vi "Drive Controller.vi"(8 "error in":errorcluster) -> ()   [LabVIEW 2018]
doc: "This VI executes continuously carrying out the current operation and responding to updates or new operation requests. It will often contain the timing or control code that is difficult to place directly in TeleOp. This VI generally opens all sensors and motors and isolates the rest of the robot code from knowing implementation details of how the operations are carried out."
uses:
  <vilib>/Rock Robotics/WPI/Framework/Completion Status.ctl
  Drive Setpoints.ctl
  Drive Operations.ctl
  <vilib>/Rock Robotics/WPI/ThirdParty/REV Robotics/SPARK MAX/Typedef/Spark MAX Control Type.ctl
  <vilib>/Rock Robotics/WPI/Gyro/WPI_GyroDevRef.ctl
  <vilib>/Rock Robotics/SystemInterfaces/AI/FPGA_AIChannel.ctl
  <vilib>/Rock Robotics/SystemInterfaces/spilib/spi_bus.ctl
  CAN Functions/SPARKMAX6Motor.ctl
  <vilib>/Rock Robotics/WPI/MotorControl/WPI_MotorControlDeviceRef.ctl
  <vilib>/Rock Robotics/WPI/MotorControl/WPI_MotorControlType.ctl
  <vilib>/Rock Robotics/SystemInterfaces/DIO/FPGA_DIOPWMChannel.ctl
  <vilib>/Rock Robotics/WPI/PWM/WPI_PWMDeadband.ctl
  <vilib>/Rock Robotics/SystemInterfaces/DIO/FPGA_DIOChannel.ctl
  <vilib>/Platform/TimedLoop/XDataNode/timing_clust.ctl
  <vilib>/Platform/TimedLoop/XDataNode/nitl_modes.ctl
  <vilib>/Platform/TimedLoop/XDataNode/wakeup.ctl
  Odometry/Typedef/Odometry.ctl
  Odometry/Typedef/Velocity Data.ctl
  <vilib>/Rock Robotics/WPI/ThirdParty/Phoenix-LabVIEW/Motor Controller/Controls/CTRE_Phoenix_MotorControl_ControlMode.ctl
  Pure Pursuit/Typedef/Pure Pursuit Telemetry.ctl
  Pure Pursuit/Typedef/Path Point.ctl
  Is High Gear.vi
  <vilib>/platform/TimedLoop/XDataNode/XDataNode.xnode
  <vilib>/Platform/TimedLoop/XDataNode/XDNodeRunTimeDep.lvlib
  <vilib>/ptbypt/NI_PtbyPt.lvlib
  Pure Pursuit/Pure Pursuit.lvlib
  <vilib>/Analysis/NI_AALPro.lvlib
panel:
  in  "Control Mode":T1
  in  "Tab Control":T2(tab)=enum."Settings"
  in  "Interactive Values":T3
  out "Setpoints":T5(graph)={"Don't move motors while reserved"=0.0, "Don't move motors while reserved"=0.0, "Left Velocity Raw"=0.0, "Right Velocity Raw"=-0.0, 0.0}
  in  "Buttons":cluster{"Execute Cmd":bool, "Abort Cmd":bool}
  out "Command Timing":cluster{"Start Time (ms)":u32, "Iterations":i32}={"Start Time (ms)"=2524017, "Iterations"=0}
  out "Status":T6
  in  "PID Constants Drivetrain":T7={"P Gain"=0.00656, "I Gain"=0.0, "D Gain"=0.01313, "F Gain"=0.005515, "I Zone"=0.0, "Min Output"=-1.0, "Max Output"=1.0} {"Max Output" min=-1.0 max=1.0 step=0.01; "Min Output" min=-1.0 max=1.0 step=0.01; "I Zone" step=0.01; "F Gain" step=0.01; "D Gain" step=0.01; "I Gain" step=0.01; "P Gain" min=0.0 step=0.01}
  in  "PIDF gains":cluster{"Kp":dbl, "Ki":dbl, "Kd":dbl, "Kf":dbl}={"Kp"=7.5, "Ki"=0.05, "Kd"=2.5, "Kf"=0.0} caption="PIDF gains (turn to angle only)" {"Kf" format="%.3f"; "Kd" format="%.5f"; "Ki" format="%.5f"; "Kp" format="%.5f"}
  in  "i Zone":dbl=8.0 format="%.2f"
  in  "Trackwidth":dbl=25.0 format="%#_13g"
  in  "Max Velocity":dbl=110.0
  in  "Max Accel":dbl=210.0
  in  "Lookahead":dbl=19.0
  in  "kffv":dbl
  in  "kffa":dbl=0.05
  in  "Velocity Offset High Gear":dbl
  in  "Velocity Offset Low Gear":dbl=0.08
  in  "Value":dbl
  in  "Run":bool
  out "Waveform Chart":dbl(graph)
  out "XY Graph":cluster{"X":dbl, "Y":dbl}[](graph)
  in  "Test":string(combo)="quasi-static ramp"
  out "Path":cluster{dbl[], dbl[]}[](graph)
  in  "Points to Follow":cluster{dbl[], dbl[]}={[0.0, 40.0, 60.0, 100.0], [0.0, 20.0, 80.0, 40.0]}
  in  "Type of Interpolation":T8(ring)=enum."Spline"
  in  "Interpolation factor (n)":i32(slide)=100 scale=0.0..20.0
  in  "Build and set Path":bool
  out "Left and Right Motor Values":T9(graph)
  out "Process Variable Vs. Setpoint":cluster{dbl, "setpoint":dbl}(graph)
  in  "PIDF gains":cluster{"Kp":dbl, "Ki":dbl, "Kd":dbl, "Kf":dbl}={"Kp"=0.06, "Ki"=0.0, "Kd"=0.0, "Kf"=0.0} {"Kf" format="%.3f"; "Kd" format="%.3f"; "Ki" format="%.3f"; "Kp" format="%.3f"}
  in  "output range 2":cluster{"output high":dbl, "output low":dbl}={"output high"=0.6, "output low"=-0.6} {"output low" format="%.2f"; "output high" format="%.2f"}
  in  "i Zone":dbl format="%.2f"
  in  "Allowed Error":dbl
  out "Current\nCmd":string="Started at  20:49:40.426\nDefault: Reserve,  L 0.0, R 0.0, D 0.000000"
  # "Click here to set min"
  # "Interactive Command: You may fill in the settings for a command\nand schedule it with the Execute button. You can observe and abort\nany command while fine tuning the code for the controller."
  # "Pure Pursuit"
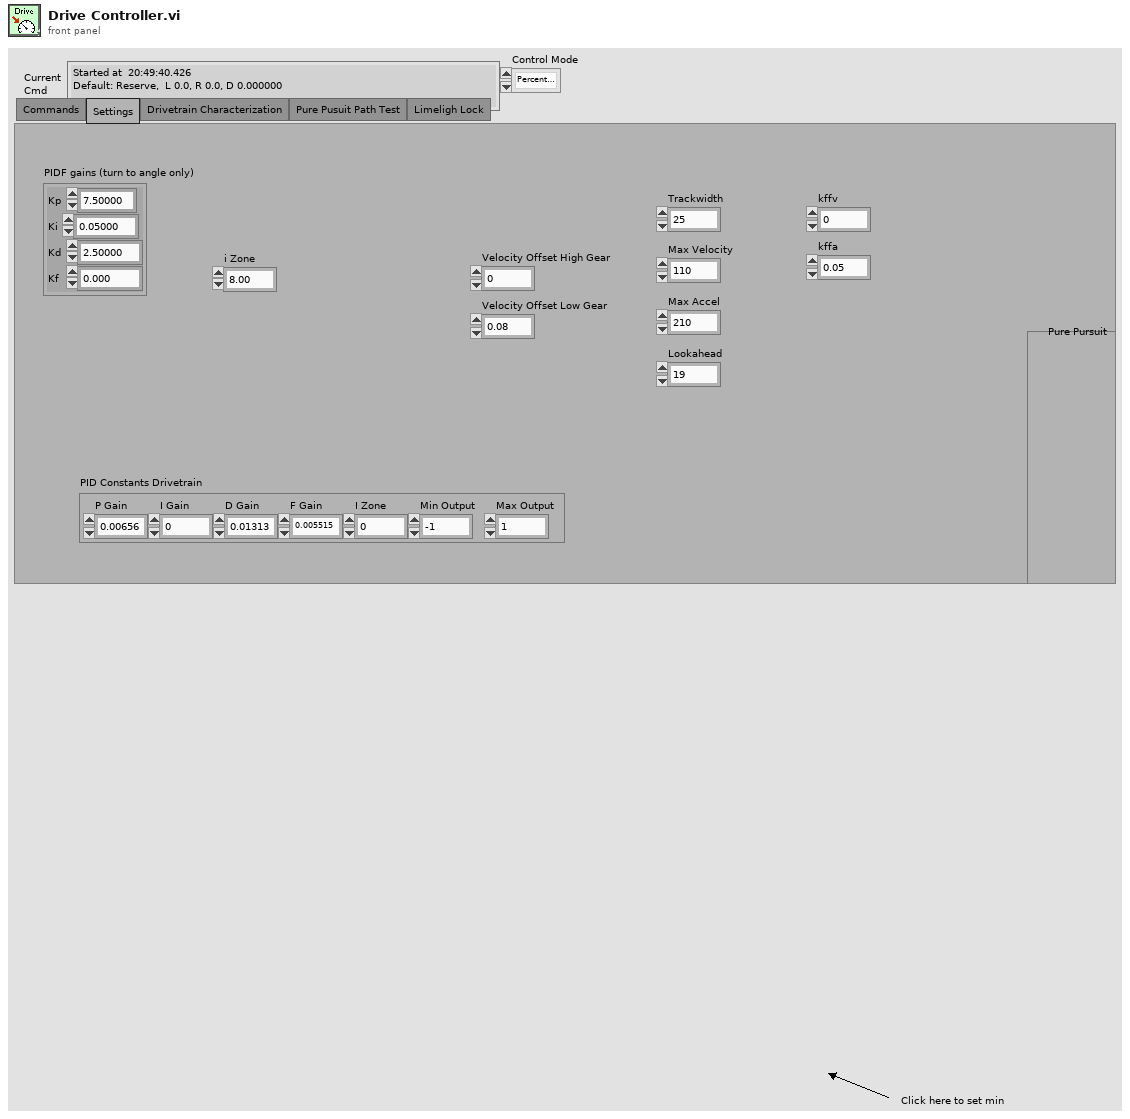
[diagram p1: front panel]
types:
  T1 = typedef "Spark MAX Control Type.ctl" = enum16{"Percent VBus", "Voltage", "Velocity", "Position", "Smart Motion", "Current", "Smart Velocity"}
  T2 = enum32{"Commands", "Settings", "Drivetrain Characterization", "Pure Pusuit Path Test", "Limeligh Lock"}
  T3 = typedef "Drive Setpoints.ctl" = cluster{"Operation":T4, "Left Setpoint":dbl, "Right Setpoint":dbl, "Duration":dbl, "Data":variant}
  T4 = typedef "Drive Operations.ctl" = enum16{"Reserve", "Read Current", "Immediate", "Drive for Time", "Drive for Distance", "Turn to Angle", "Drivetrain Char", "Pure Pursuit", "Limelight Lock"}
  T5 = cluster{"Don't move motors while reserved":dbl, "Don't move motors while reserved":dbl, "Left Velocity Raw":sgl, "Right Velocity Raw":sgl, sgl}
  T6 = typedef "Completion Status.ctl" = enum16{"Successful", "Aborted", "Incomplete"}
  T7 = cluster{"P Gain":dbl, "I Gain":dbl, "D Gain":dbl, "F Gain":dbl, "I Zone":dbl, "Min Output":dbl, "Max Output":dbl}
  T8 = enum16{"Linear", "Polynomial", "Spline", "Rational"}
  T9 = cluster{"Left Motor Value":dbl, "Right Motor Value":dbl}
  T10 = typedef "WPI_GyroDevRef.ctl" = cluster{"DevStatus":errorcluster, "Analog Channel":T11, "Gain (VoltsPerDegree/Second)":dbl, "Gyro Type":enum16{"Analog", "XRS450"}, "Handle":i32, "SPI Bus":T12, "Device Found":bool, "Sample Rate":dbl, "Calibrate On Open":bool, "Offset":dbl}
  T11 = typedef "FPGA_AIChannel.ctl" = enum8{"AI 0", "AI 1", "AI 2", "AI 3", "AI MXP 0", "AI MXP 1", "AI MXP 2", "AI MXP 3", "Invalid"}
  T12 = typedef "spi_bus.ctl" = enum16{"SPI On-Board, CS0", "SPI On-Board, CS1", "SPI On-Board, CS2", "SPI On-Board, CS3", "SPI MXP", "Invalid"}
  T13 = typedef "SPARKMAX6Motor.ctl" = cluster{"FrontLeftMaster":T14, "FrontLeftSlave1":T14, "FrontLeftSlave2":T14, "FrontRightMaster":T14, "FrontRightSlave1":T14, "FrontRightSlave2":T14}
  T14 = typedef "WPI_MotorControlDeviceRef.ctl" = cluster{"DeviceStatus":errorcluster, "Type":T15, "PWM":cluster{"PWM Channel":T16, "DeadBand":T17}, "CAN":cluster{"Device Number":u8, "SetOutput VI Ref":variant, "GetOutput VI Ref":variant, "Enable VI Ref":variant, "Disable VI Ref":variant, "Data":variant}, "Invert":bool, "DIO PWM":cluster{"PWM \"Enable\" Channel":T16, "DIOChannel":T18, "PWM Rate":dbl}}
  T15 = typedef "WPI_MotorControlType.ctl" = enum16{"PWM", "CAN", "DIO PWM"}
  T16 = typedef "FPGA_DIOPWMChannel.ctl" = enum8{"PWM 0", "PWM 1", "PWM 2", "PWM 3", "PWM 4", "PWM 5", "PWM 6", "PWM 7", "PWM 8", "PWM 9", "PWM MXP 0", "PWM MXP 1", "PWM MXP 2", "PWM MXP 3", "PWM MXP 4", "PWM MXP 5", "PWM MXP 6", "PWM MXP 7", "PWM MXP 8", "PWM MXP 9", "Invalid"}
  T17 = typedef "WPI_PWMDeadband.ctl" = cluster{"Name":string, "maxPositivePwm":i32, "minPositivePwm":i32, "centerPwm":i32, "maxNegativePwm":i32, "minNegativePwm":i32, "angularRange":u16}
  T18 = typedef "FPGA_DIOChannel.ctl" = enum8{"DIO 0", "DIO 1", "DIO 2", "DIO 3", "DIO 4", "DIO 5", "DIO 6", "DIO 7", "DIO 8", "DIO 9", "DIO MXP 0", "DIO MXP 1", "DIO MXP 2", "DIO MXP 3", "DIO MXP 4", "DIO MXP 5", "DIO MXP 6", "DIO MXP 7", "DIO MXP 8", "DIO MXP 9", "DIO MXP 10", "DIO MXP 11", "DIO MXP 12", "DIO MXP 13", "DIO MXP 14", "DIO MXP 15", "SPI Port CS1", "SPI Port CS2", "SPI Port CS3", "SPI Port MISO", "SPI Port MOSI", "Invalid"}
  T19 = typedef "XDNodeRunTimeDep.lvlib/timing_clust.ctl" = cluster{"Expected End [f-1]":u64, "Actual End [f-1]":u64, "Finished Late? [f-1]":bool, "Expected End [i-1]":u64, "Actual End [i-1]":u64, "Finished Late? [i-1]":bool, "Expected Start [i]":u64, "Actual Start [i]":u64, "Expected Start [f]":u64, "Actual Start [f]":u64, "Source Name":string, "Structure Name":string, "Period":i64, "Deadline":i64, "Offset":i64, "Start":i64, "Priority":i32, "Timeout":i32, "Mode":T20, "Wakeup Reason":T21, "Error":errorcluster, "Source Type":string, "Secondary Source Type":string, "Global End Time":u64, "Global Start Time":u64, "Frame Duration":u64, "Iteration Duration":u64, "Assigned CPU":i32, "I/O Scan Engine Mode":u32}
  T20 = typedef "XDNodeRunTimeDep.lvlib/nitl_modes.ctl" = enum32{"No Change", "Process missed periods, maintain original phase", "Discard missed periods, maintain original phase", "Process missed periods, ignore original phase", "Discard missed periods, ignore original phase"}
  T21 = typedef "XDNodeRunTimeDep.lvlib/wakeup.ctl" = enum32{"Normal", "Aborted", "Asynchronous wakeup", "Timing source error", "Timed loop error", "Timeout"}
  T22 = typedef "Command Status Info.ctl" = cluster{"Name":string, "Status":T6, "notifier out":T23}
  T23 = typedef "Completion Notifier.ctl" = refnum<notifier>
  T24 = cluster{"SubSystem Data":T3, cluster{"Start Time (ms)":u32, "Iterations":i32}, cluster{"Command Info":T22, "Description":string, "Default Command":T3, "queue out":refnum<queue>, "Subsystem Name":string}}
  T25 = typedef "Pure Pursuit.lvlib/Pure Pursuit Telemetry.ctl" = cluster{"Target Point":T26, "Close Point":T26, "Curvature":dbl, "index out":i32}
  T26 = typedef "Pure Pursuit.lvlib/Path Point.ctl" = cluster{"x":dbl, "y":dbl, "heading":dbl, "curvature":dbl, "total distance":dbl, "velocity expected":dbl}
  T27 = typedef "Odometry.ctl" = cluster{"x":dbl, "y":dbl, "theta":dbl, "Left Encoder":dbl, "Right Encoder":dbl, "Late Iterations":i16}
  T28 = typedef "CTRE_Phoenix_MotorControl_ControlMode.ctl" = u16
  T29 = typedef "Velocity Data.ctl" = cluster{"Right Velocity Raw":sgl, "Left Velocity Raw":sgl}
  T30 = cluster{"SubSystem Data":T3, cluster{"Start Time (ms)":u32, "Iterations":i32}, "Default Command Arguments":cluster{"Command Info":T22, "Description":string, "Default Command":T3, "queue out":refnum<queue>, "Subsystem Name":string}}
  T31 = cluster{"P Gain":bool, "I Gain":bool, "D Gain":bool, "F Gain":bool, "I Zone":bool, "Min Output":bool, "Max Output":bool}
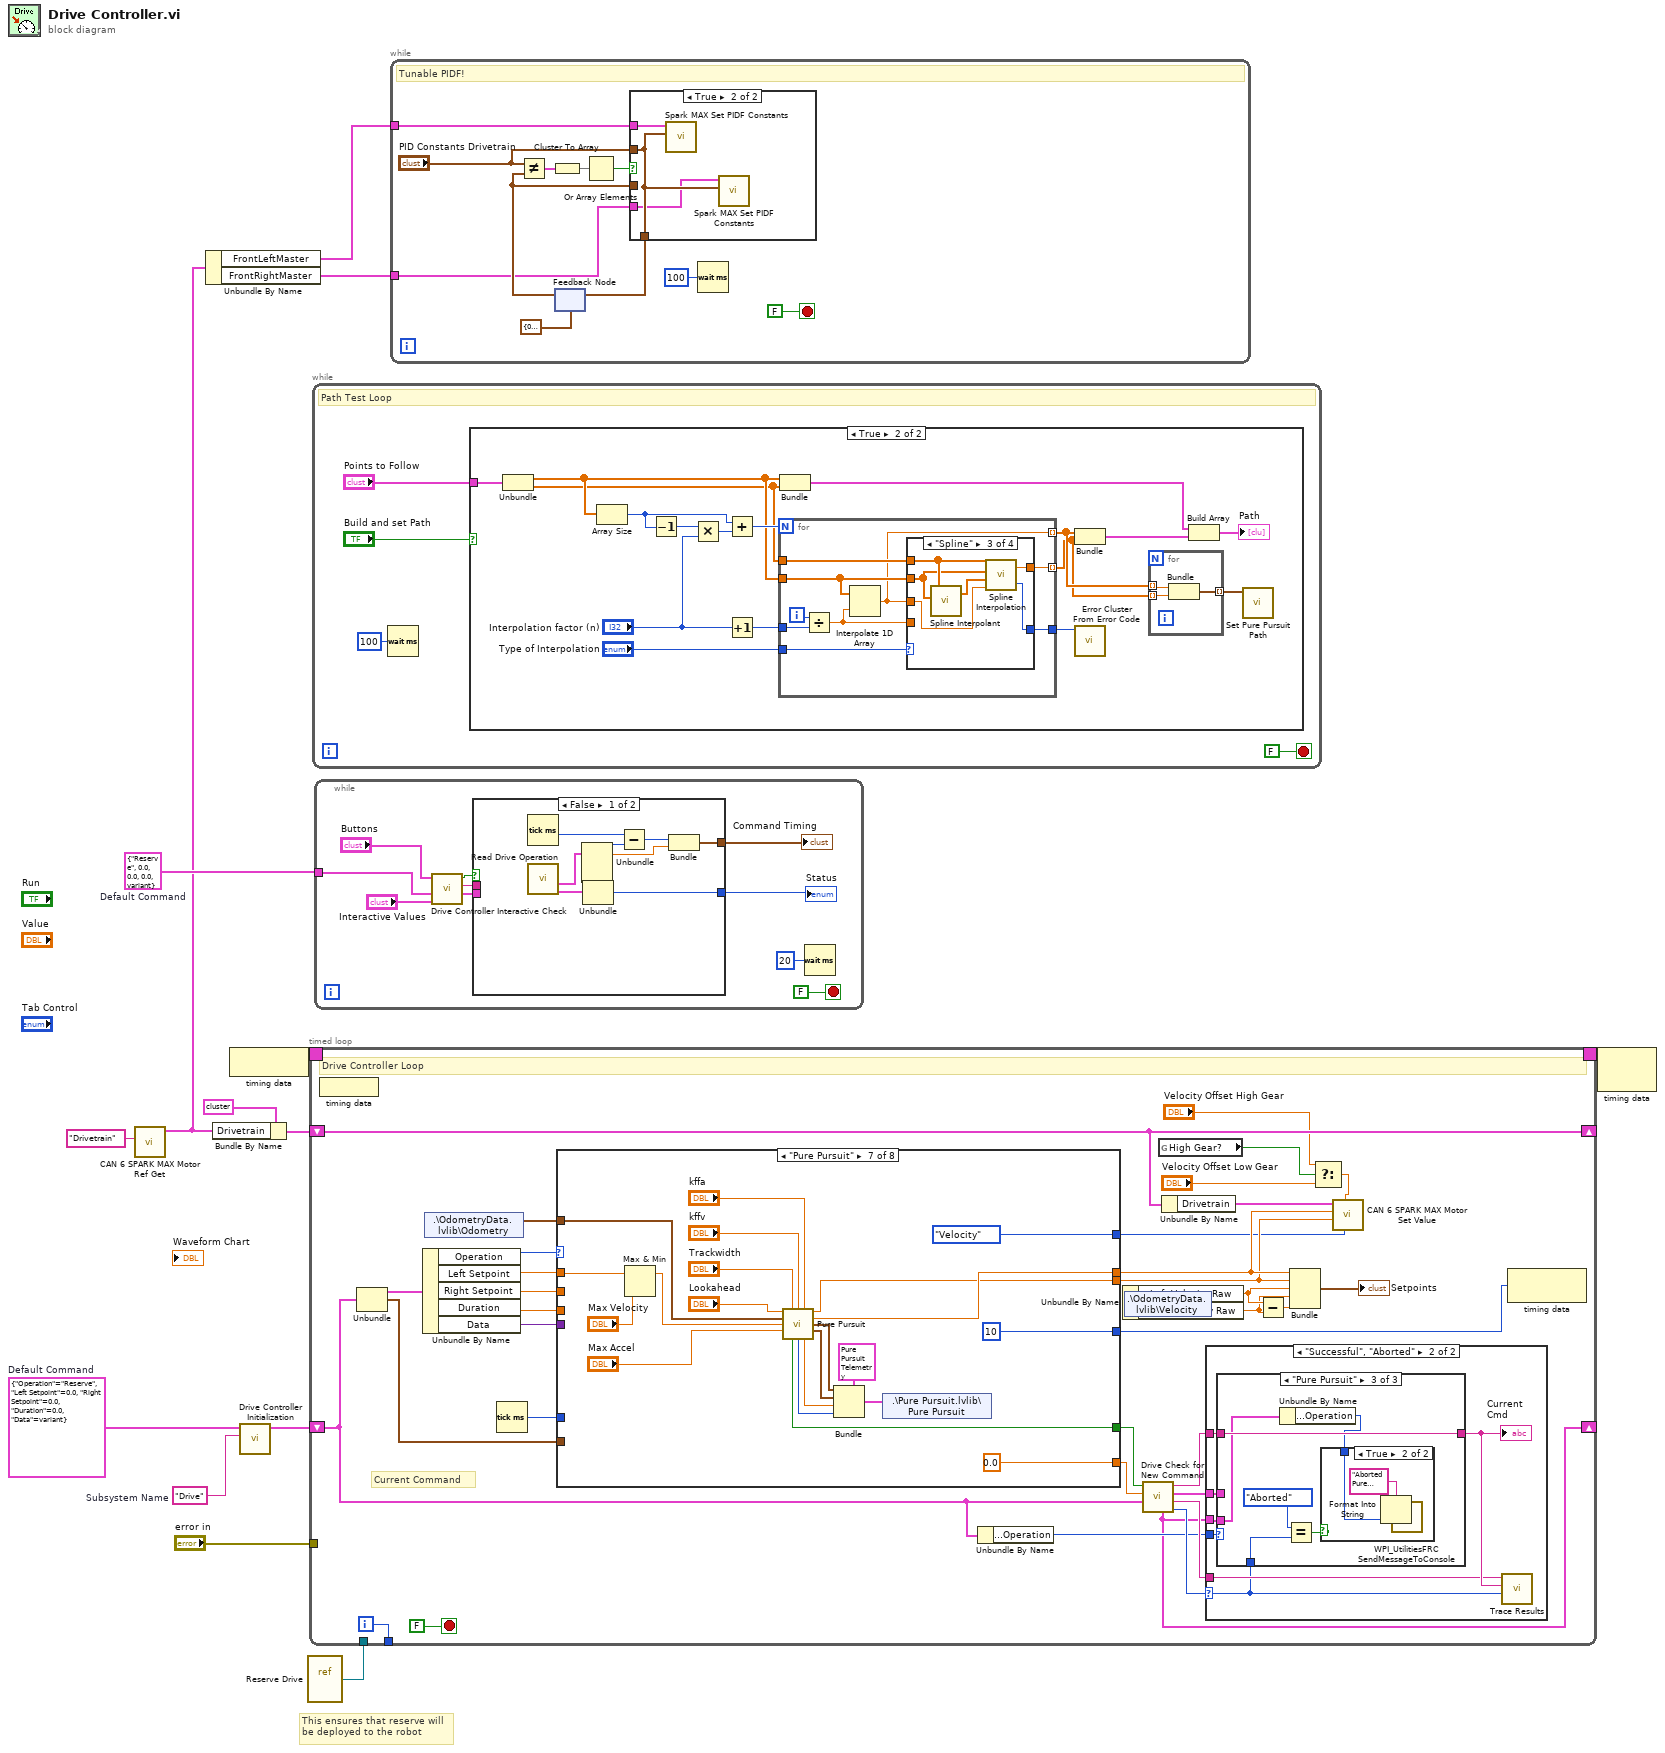
[diagram p0: block diagram]
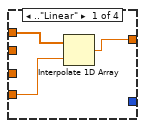
[diagram p4: hidden frame]
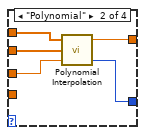
[diagram p5: hidden frame]
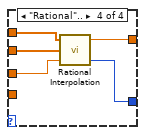
[diagram p6: hidden frame]
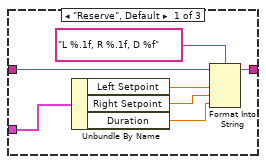
[diagram p8: hidden frame]
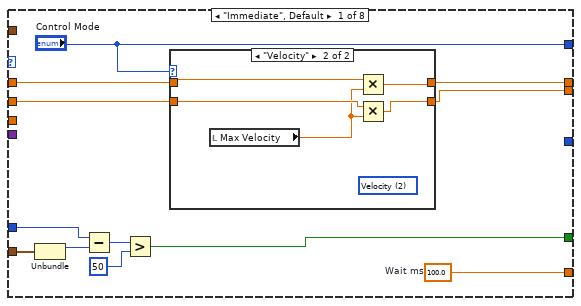
[diagram p11: hidden frame]
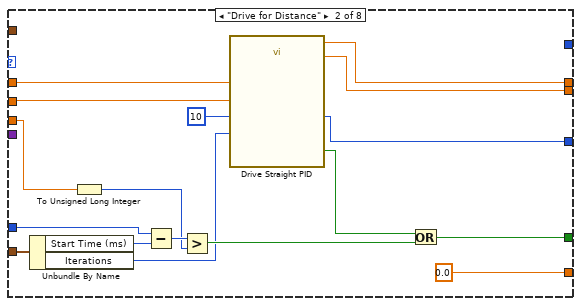
[diagram p13: hidden frame]
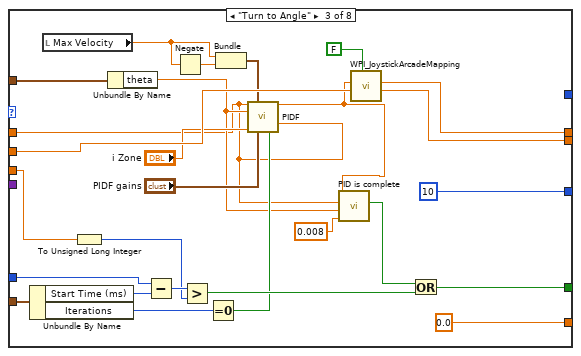
[diagram p14: hidden frame]
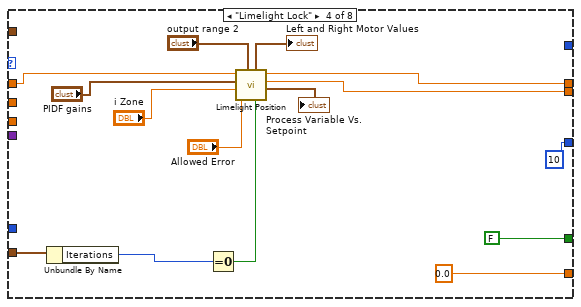
[diagram p15: hidden frame]
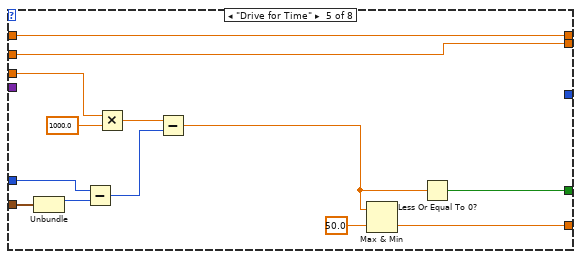
[diagram p16: hidden frame]
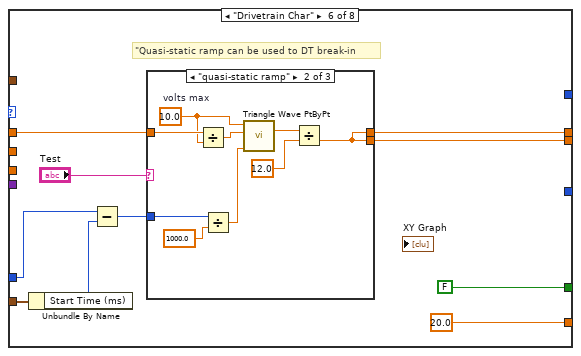
[diagram p17: hidden frame]
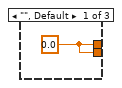
[diagram p18: hidden frame]
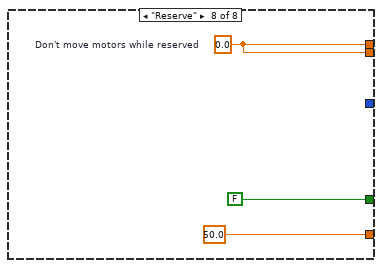
[diagram p20: hidden frame]
diagram:
  w7 = T3 {"Operation"=enum."Reserve", "Left Setpoint"=0.0, "Right Setpoint"=0.0, "Duration"=0.0, "Data"=variant}  # Default Command
  w10 = T3 {"Operation"=enum."Reserve", "Left Setpoint"=0.0, "Right Setpoint"=0.0, "Duration"=0.0, "Data"=variant}  # Default Command
  w14 = "Drive"  # Subsystem Name
  # "This ensures that reserve will\nbe deployed to the robot"
  n1 = call "CAN 6 SPARK MAX Motor Ref Get.vi"("refnum name"="Drivetrain") -> ("TalonSRX6MotorRef out"=w3:T13)  [unwired: 9 in, 1 out]
  n2 = Unbundle By Name(w3) -> ("FrontLeftMaster"=w2:T14, "FrontRightMaster"=w1:T14)
  n3 = Bundle By Name(cluster=cluster{"Gyro":T10, "Drivetrain":T13} {"Gyro"={"DevStatus"={"status"=FALSE, "code"=0, "source"=""}, "Analog Channel"=enum."Invalid", "Gain (VoltsPerDegree/Second)"=0.0, "Gyro Type"=enum."Analog", "Handle"=0, "SPI Bus"=enum."Invalid", "Device Found"=FALSE, "Sample Rate"=1.0, "Calibrate On Open"=FALSE, "Offset"=0.0}, "Drivetrain"={"FrontLeftMaster"={"DeviceStatus"={"status"=FALSE, "code"=0, "source"=""}, "Type"=enum."PWM", "PWM"={"PWM Channel"=enum."PWM 1", "DeadBand"={"Name"="", "maxPositivePwm"=0, "minPositivePwm"=0, "centerPwm"=0, "maxNegativePwm"=0, "minNegativePwm"=0, "angularRange"=0}}, "CAN"={"Device Number"=0, "SetOutput VI Ref"=variant(enum8{"Percent VBus", "Current", "Speed", "Position", "Voltage"} enum."Percent VBus"), "GetOutput VI Ref"=variant(refnum<k1> refnum), "Enable VI Ref"=variant(dbl 12.0), "Disable VI Ref"=variant(enum8{"Percent VBus", "Speed", "Position", "Slave", "Unchanged / Invalid", "Voltage Compensation", "Current", "Motion Profile"} enum."Percent VBus"), "Data"=variant}, "Invert"=FALSE, "DIO PWM"={"PWM \"Enable\" Channel"=enum."Invalid", "DIOChannel"=enum."Invalid", "PWM Rate"=0.0}}, "FrontLeftSlave1"={"DeviceStatus"={"status"=FALSE, "code"=0, "source"=""}, "Type"=enum."PWM", "PWM"={"PWM Channel"=enum."PWM 1", "DeadBand"={"Name"="", "maxPositivePwm"=0, "minPositivePwm"=0, "centerPwm"=0, "maxNegativePwm"=0, "minNegativePwm"=0, "angularRange"=0}}, "CAN"={"Device Number"=0, "SetOutput VI Ref"=variant(enum8{"Percent VBus", "Current", "Speed", "Position", "Voltage"} enum."Percent VBus"), "GetOutput VI Ref"=variant(refnum<k1> refnum), "Enable VI Ref"=variant(dbl 12.0), "Disable VI Ref"=variant(enum8{"Percent VBus", "Speed", "Position", "Slave", "Unchanged / Invalid", "Voltage Compensation", "Current", "Motion Profile"} enum."Percent VBus"), "Data"=variant}, "Invert"=FALSE, "DIO PWM"={"PWM \"Enable\" Channel"=enum."Invalid", "DIOChannel"=enum."Invalid", "PWM Rate"=0.0}}, "FrontLeftSlave2"={"DeviceStatus"={"status"=FALSE, "code"=0, "source"=""}, "Type"=enum."PWM", "PWM"={"PWM Channel"=enum."PWM 1", "DeadBand"={"Name"="", "maxPositivePwm"=0, "minPositivePwm"=0, "centerPwm"=0, "maxNegativePwm"=0, "minNegativePwm"=0, "angularRange"=0}}, "CAN"={"Device Number"=0, "SetOutput VI Ref"=variant(enum8{"Percent VBus", "Current", "Speed", "Position", "Voltage"} enum."Percent VBus"), "GetOutput VI Ref"=variant(refnum<k1> refnum), "Enable VI Ref"=variant(dbl 12.0), "Disable VI Ref"=variant(enum8{"Percent VBus", "Speed", "Position", "Slave", "Unchanged / Invalid", "Voltage Compensation", "Current", "Motion Profile"} enum."Percent VBus"), "Data"=variant}, "Invert"=FALSE, "DIO PWM"={"PWM \"Enable\" Channel"=enum."Invalid", "DIOChannel"=enum."Invalid", "PWM Rate"=0.0}}, "FrontRightMaster"={"DeviceStatus"={"status"=FALSE, "code"=0, "source"=""}, "Type"=enum."PWM", "PWM"={"PWM Channel"=enum."PWM 1", "DeadBand"={"Name"="", "maxPositivePwm"=0, "minPositivePwm"=0, "centerPwm"=0, "maxNegativePwm"=0, "minNegativePwm"=0, "angularRange"=0}}, "CAN"={"Device Number"=0, "SetOutput VI Ref"=variant(enum8{"Percent VBus", "Current", "Speed", "Position", "Voltage"} enum."Percent VBus"), "GetOutput VI Ref"=variant(refnum<k1> refnum), "Enable VI Ref"=variant(dbl 12.0), "Disable VI Ref"=variant(enum8{"Percent VBus", "Speed", "Position", "Slave", "Unchanged / Invalid", "Voltage Compensation", "Current", "Motion Profile"} enum."Percent VBus"), "Data"=variant}, "Invert"=FALSE, "DIO PWM"={"PWM \"Enable\" Channel"=enum."Invalid", "DIOChannel"=enum."Invalid", "PWM Rate"=0.0}}, "FrontRightSlave1"={"DeviceStatus"={"status"=FALSE, "code"=0, "source"=""}, "Type"=enum."PWM", "PWM"={"PWM Channel"=enum."PWM 1", "DeadBand"={"Name"="", "maxPositivePwm"=0, "minPositivePwm"=0, "centerPwm"=0, "maxNegativePwm"=0, "minNegativePwm"=0, "angularRange"=0}}, "CAN"={"Device Number"=0, "SetOutput VI Ref"=variant(enum8{"Percent VBus", "Current", "Speed", "Position", "Voltage"} enum."Percent VBus"), "GetOutput VI Ref"=variant(refnum<k1> refnum), "Enable VI Ref"=variant(dbl 12.0), "Disable VI Ref"=variant(enum8{"Percent VBus", "Speed", "Position", "Slave", "Unchanged / Invalid", "Voltage Compensation", "Current", "Motion Profile"} enum."Percent VBus"), "Data"=variant}, "Invert"=FALSE, "DIO PWM"={"PWM \"Enable\" Channel"=enum."Invalid", "DIOChannel"=enum."Invalid", "PWM Rate"=0.0}}, "FrontRightSlave2"={"DeviceStatus"={"status"=FALSE, "code"=0, "source"=""}, "Type"=enum."PWM", "PWM"={"PWM Channel"=enum."PWM 1", "DeadBand"={"Name"="", "maxPositivePwm"=0, "minPositivePwm"=0, "centerPwm"=0, "maxNegativePwm"=0, "minNegativePwm"=0, "angularRange"=0}}, "CAN"={"Device Number"=0, "SetOutput VI Ref"=variant(enum8{"Percent VBus", "Current", "Speed", "Position", "Voltage"} enum."Percent VBus"), "GetOutput VI Ref"=variant(refnum<k1> refnum), "Enable VI Ref"=variant(dbl 12.0), "Disable VI Ref"=variant(enum8{"Percent VBus", "Speed", "Position", "Slave", "Unchanged / Invalid", "Voltage Compensation", "Current", "Motion Profile"} enum."Percent VBus"), "Data"=variant}, "Invert"=FALSE, "DIO PWM"={"PWM \"Enable\" Channel"=enum."Invalid", "DIOChannel"=enum."Invalid", "PWM Rate"=0.0}}}}, "Drivetrain"=w3) -> (w5:cluster{"Gyro":T10, "Drivetrain":T13})
  n4 = node-c288() -> (w9:T19)
  n5 = call "Drive Controller Initialization.vi"("Subsystem Name"=w14, "Default Command"=w10) -> ("Current Command"=w12:T24)  [unwired: 9 in]
  n6 = vi-ref "Reserve Drive.vi"() -> (w11:refnum<vi>)
  n7 = timed-loop {
    shift-right: [w24] -> _
    shift-left: w12 -> [w33]
    tunnel: [w48] -> _
    tunnel: "error in" -> [_]
    tunnel: w11 -> [_]
    timing: w9 -> [_]
    timing-out: [_] -> w8
    shift-right: [w31] -> _
    shift-left: w5 -> [w31]
    i -> [w48]
    stop <- FALSE stop-if-true
    # "Current Command"
    # "Drive Controller Loop"
    n8 = node-c288() -> ()  [unwired: 1 in]
    n9 = Unbundle(w33) -> ("SubSystem Data"=w47:T3, w36:cluster{"Start Time (ms)":u32, "Iterations":i32})  [unwired: 1 out]
    n10 = Unbundle By Name(w47) -> ("Operation"=w46:T4, "Left Setpoint"=w45:dbl, "Right Setpoint"=w44:dbl, "Duration"=w43:dbl, "Data"=w25:variant)
    n11 = shared-variable ".\\OdometryData.lvlib\\Odometry"() -> (w26:T27)  [unwired: 1 in, 1 out]
    n12 = Tick Count (ms)() -> (millisecond timer value=w42:u32)
    n13 = case shown="\"Pure Pursuit\"" w46 {
      tunnel: [w89 0.0 ("Wait ms") 0.0 ("Wait ms") 0.0 ("Wait ms") w156 20.0 ("Wait ms") 0.0 ("Wait ms") 50.0] -> w35
      tunnel: [w84 w104 w134 FALSE w162 FALSE ("ignore previous (F)") w208 FALSE ("ignore previous (F)")] -> w40
      tunnel: w36 -> [w83 w111 w138 w153 w164 w173 _ _]
      tunnel: [w80 w108 w122 w144 w161 w176 w197 w210] -> w30
      tunnel: [w79 w107 w120 w143 w160 w175 w196 w210] -> w29
      tunnel: w45 -> [w82 w103 w114 w147 w161 w174 w195 _]
      tunnel: w44 -> [w81 w102 w121 _ w160 _ _ _]
      tunnel: w43 -> [_ w99 w132 _ w155 _ _ _]
      tunnel: w42 -> [w85 w110 w137 _ w159 w171 _ _]
      tunnel: [_ w100 i64 10 ("Period") i64 10 ("Period") _ _ i64 10 ("Period") _] -> w34
      tunnel: w26 -> [_ _ w126 _ _ _ w205 _]
      tunnel: w25 -> [_ _ _ _ _ _ _ _]
      tunnel: ["Control Mode" _ _ _ _ _ Spark_MAX_Control_Type."Velocity" ("Control Mode") _] -> w15
      frame "Immediate", Default {
        w89 = 100.0  # Wait ms
        n14 = Unbundle(w83) -> ("Start Time (ms)"=w86:u32)  [unwired: 1 out]
        n15 = Subtract(x=w85, y=w86) -> (x-y=w87:u32)
        n16 = Greater?(x=w87, y=u32 50 ("Left Motor")) -> (0:w84:bool)
        n17 = case shown="\"Velocity\"" "Control Mode" {
          tunnel: w82 -> [w91 w96]
          tunnel: w81 -> [w90 w94]
          tunnel: [w91 w95] -> w80
          tunnel: [w90 w93] -> w79
          frame "Percent VBus", Default {
          }
          frame "Velocity" {
            (unwired) T28 2 items=["PercentOutput"=0, "Position"=1, "Velocity"=2, "Current"=3, "Follower"=5, "MotionProfile"=6, "MotionMagic"=7, "MotionMagicArc"=8, "MotionProfileArc"=10, "Disabled"=15] ("Control Mode")
            n18 = local read "Max Velocity"() -> (w92:dbl)
            n19 = Multiply(x=w96, y=w92) -> (x*y=w95:dbl)
            n20 = Multiply(x=w94, y=w92) -> (x*y=w93:dbl)
          }
        }
      }
      frame "Drive for Distance" {
        w100 = i64 10 ("Period")
        n21 = Unbundle By Name(w111) -> ("Start Time (ms)"=w98:u32, "Iterations"=w101:i32)
        n22 = To Unsigned Long Integer(number=w99) -> (unsigned 32bit integer=w97:u32)
        n23 = Subtract(x=w110, y=w98) -> (x-y=w109:u32)
        n24 = Greater?(x=w109, y=w97) -> (0:w105:bool)
        n25 = call "Drive Straight PID.vi"("Angle Offset"=w102, "Iteration"=w101, "target distance"=w103, "Period (ms)"=w100) -> ("Complete?"=w106:bool, "Right Axis"=w107:dbl, "Left Axis"=w108:dbl)  [unwired: 5 in]
        n26 = Or(x=w106, y=w105) -> (x .or. y?=w104:bool)
      }
      frame "Turn to Angle" {
        n27 = Unbundle By Name(w138) -> ("Start Time (ms)"=w131:u32, "Iterations"=w129:i32)
        n28 = local read "Max Velocity"() -> (w125:dbl)
        n29 = To Unsigned Long Integer(number=w132) -> (unsigned 32bit integer=w130:u32)
        n30 = Unbundle By Name(w126) -> ("theta"=w115:dbl)
        n31 = Subtract(x=w137, y=w131) -> (x-y=w136:u32)
        n32 = Negate(x=w125) -> (-x=w124:dbl)
        n33 = Greater?(x=w136, y=w130) -> (0:w135:bool)
        n34 = Equal To 0?(x=w129) -> (x = 0?=w118:bool)
        n35 = Bundle("Max Velocity"=w125, w124) -> (w117:cluster{"Max Velocity":dbl, dbl})  [unwired: 1 in]
        n36 = call "PIDF.vi"("setpoint"=w114, "output range"=w117, "process variable"=w115, "Feedforward"=w114, "i Zone"="i Zone", "PIDF gains"="PIDF gains", "reinitialize? (F)"=w118) -> ("output"=w113:dbl)  [unwired: 6 in, 2 out]
        n37 = call "PID is complete.vi"("threshold"=0.008, "process variable"=w115, "setpoint"=w114, "PID Output"=w113) -> ("PID is Done?"=w128:bool)  [unwired: 6 in, 1 out]
        n38 = call <vilib>:"WPI_JoystickArcadeMapping.vi"("Square Inputs"=FALSE, "Y axis value"=w121, "X axis value"=w113) -> ("Right Motor Value"=w120:dbl, "Left Motor Value"=w122:dbl)  [unwired: 7 in]
        n39 = Or(x=w128, y=w135) -> (x .or. y?=w134:bool)
      }
      frame "Limelight Lock" {
        n40 = Unbundle By Name(w153) -> ("Iterations"=w151:i32)
        n41 = Equal To 0?(x=w151) -> (x = 0?=w148:bool)
        n42 = call "Limelight Position.vi"("Boolean"=w148, "Allowed Error"="Allowed Error", "output range in"="output range 2", "i Zone"="i Zone", "PIDF gains"="PIDF gains", "Left Setpoint"=w147) -> ("Process Variable Vs. Setpoint"=→"Process Variable Vs. Setpoint":cluster{dbl, "setpoint":dbl}, "Right Motor Value"=w143:dbl, "Left Motor Value"=w144:dbl, "Left and Right Motor Values"=→"Left and Right Motor Values":T9)  [unwired: 2 in]
      }
      frame "Drive for Time" {
        n43 = Unbundle(w164) -> ("Start Time (ms)"=w163:u32)  [unwired: 1 out]
        n44 = Subtract(x=w159, y=w163) -> (x-y=w167:u32)
        n45 = Multiply(x=w155, y=1000.0) -> (x*y=w166:dbl)
        n46 = Subtract(x=w166, y=w167) -> (x-y=w158:dbl)
        n47 = Max & Min(x=w158, y=50.0) -> (min(x,y)=w156:dbl)  [unwired: 1 out]
        n48 = Less Or Equal To 0?(x=w158) -> (x <= 0?=w162:bool)
      }
      frame "Drivetrain Char" {
        # "\"Quasi-static ramp can be used to DT break-in"
        n49 = Unbundle By Name(w173) -> ("Start Time (ms)"=w172:u32)
        n50 = Subtract(x=w171, y=w172) -> (x-y=w170:u32)
        n51 = case shown="\"quasi-static ramp\"" "Test" {
          tunnel: [w178 w181 w188] -> w176
          tunnel: [w178 w181 w188] -> w175
          tunnel: w174 -> [_ w183 w188]
          tunnel: w170 -> [_ w187 _]
          frame "", Default {
            w178 = 0.0
          }
          frame "quasi-static ramp" {
            w180 = 10.0  # volts max
            n52 = Divide(x=w183, y=w180) -> (x/y=w184:dbl)
            n53 = Divide(x=w187, y=1000.0 ("amplitude")) -> (x/y=w186:dbl)
            n54 = call <vilib>:"Triangle Wave PtByPt.vi"("time"=w186, "frequency"=w184, "amplitude"=w180) -> ("triangle wave"=w182:dbl)  [unwired: 1 in]
            n55 = Divide(x=w182, y=12.0) -> (x/y=w181:dbl)
          }
          frame "step-voltage acceleration" {
          }
        }
      }
      frame "Pure Pursuit" {
        n56 = Max & Min(x=w195, y="Max Velocity") -> (max(x,y)=w193:dbl)  [unwired: 1 out]
        n57 = call "Pure Pursuit.vi"("Lookahead"="Lookahead", "Trackwidth"="Trackwidth", "kffv"="kffv", "kffa"="kffa", "Odometry"=w205, "Max Velocity"=w193, "Max Accel"="Max Accel") -> ("Left Velocity"=w196:dbl, "Right Velocity"=w197:dbl, "Target Point"=w202:T26, "Close Point"=w201:T26, "Finished?"=w208:bool, "index out"=w190:i32, "Curvature"=w200:dbl)  [unwired: 1 in, 1 out]
        n58 = Bundle(cluster=T25 {"Target Point"={"x"=0.0, "y"=0.0, "heading"=0.0, "curvature"=0.0, "total distance"=0.0, "velocity expected"=0.0}, "Close Point"={"x"=0.0, "y"=0.0, "heading"=0.0, "curvature"=0.0, "total distance"=0.0, "velocity expected"=0.0}, "Curvature"=0.0, "index out"=0} ("Pure Pursuit"), "Target Point"=w202, "Close Point"=w201, "Curvature"=w200, "index out"=w190) -> (w191:T25)
        n59 = shared-variable ".\\Pure Pursuit.lvlib\\Pure Pursuit"(w191) -> ()  [unwired: 1 in, 1 out]
      }
      frame "Reserve" {
        w210 = 0.0  # Don't move motors while reserved
      }
    }
    n60 = Unbundle By Name(w33) -> ("SubSystem Data.Operation"=w32:T4)
    n61 = shared-variable ".\\OdometryData.lvlib\\Velocity"() -> (w19:T29)  [unwired: 1 in, 1 out]
    n62 = Unbundle By Name(w19) -> ("Left Velocity Raw"=w18:sgl, "Right Velocity Raw"=w17:sgl)
    n63 = call "Drive Check for New Command.vi"("input cluster"=w33, "Wait time (ms)"=w35, "Finished?"=w40) -> ("Completion"=w41:T6, "Subsystem Name"=w37:string, "Current Command"=w38:T3, "Initial Trace String"=w39:string, "Next Command"=w24:T30)  [unwired: 4 in]
    n64 = global read "Is High Gear.vi" "High Gear?"() -> (w22:bool)
    n65 = Unbundle By Name(w31) -> ("Drivetrain"=w27:T13)
    n66 = case shown="\"Successful\", \"Aborted\"" w41 {
      selector: w41 -> [_ w55]
      tunnel: w39 -> [_ w59]
      tunnel: w38 -> [_ w60]
      tunnel: w37 -> [_ w57]
      tunnel: w32 -> [_ w56]
      tunnel: w24 -> [_ w54]
      frame "Incomplete", Default {
        # "Continuing current command"
      }
      frame "Successful", "Aborted" {
        # "Report and setup for next command"
        n67 = case shown="\"Pure Pursuit\"" w56 {
          tunnel: w60 -> [w64 _ _]
          tunnel: w59 -> [w63 w68 w74]
          tunnel: [w62 w68 w74] -> w58
          tunnel: w55 -> [_ _ w73]
          tunnel: w54 -> [_ _ w70]
          frame "Reserve", Default {
            n68 = Unbundle By Name(w64) -> ("Left Setpoint"=w66:dbl, "Right Setpoint"=w67:dbl, "Duration"=w61:dbl)
            n69 = Format Into String(format string="L %.1f, R %.1f, D %f", initial string=w63, w66, w67, w61) -> (resulting string=w62:string)  [unwired: 1 in, 1 out]
          }
          frame "Read Current" {
            # "Placeholder for \ncomplex commands\nwith cleanup"
          }
          frame "Pure Pursuit" {
            n70 = Unbundle By Name(w70) -> ("SubSystem Data.Operation"=w69:T4)
            n71 = Equal?(x=Completion_Status."Aborted", y=w73) -> (x = y?=w71:bool)
            n72 = case shown="True" w71 {
              tunnel: w69 -> [_ w75]
              frame False {
              }
              frame True {
                n73 = Format Into String(format string="Aborted Pure Pursuit for: %s", w75) -> (resulting string=w77:string)  [unwired: 2 in, 1 out]
                n74 = call <vilib>:"WPI_UtilitiesFRC SendMessageToConsole.vi"("Message"=w77) -> ()  [unwired: 14 in, 1 out]
              }
            }
          }
        }
        "Current\nCmd" <- w58
        n75 = call <vilib>:"Trace Results.vi"("Status of previous command"=w55, "Description"=w58, "Subsystem"=w57) -> ()  [unwired: 9 in]
      }
    }
    n76 = Subtract(x=w18, y=w17) -> (x-y=w16:sgl)
    n77 = Bundle("Don't move motors while reserved"=w30, "Don't move motors while reserved"=w29, "Left Velocity Raw"=w18, "Right Velocity Raw"=w17, w16) -> (→"Setpoints":T5)  [unwired: 1 in]
    n78 = Select(t="Velocity Offset High Gear", s=w22, f="Velocity Offset Low Gear") -> (s? t:f=w20:dbl)
    n79 = call "CAN 6 SPARK MAX Motor Set Value.vi"("Control Mode"=w15, "Velocity Offset"=w20, "Right Power"=w29, "Left Power"=w30, "Drivetrain"=w27) -> ()  [unwired: 7 in]
    n80 = node-c288(w34) -> ()  [unwired: 1 out]
  }
  n81 = while {
    stop <- FALSE stop-if-true
    # "Path Test Loop"
    n82 = Wait (ms)(milliseconds to wait=u32 100) -> ()  [unwired: 1 out]
    n83 = case shown="True" "Build and set Path" {
      tunnel: "Points to Follow" -> [_ w225]
      frame False {
      }
      frame True {
        n84 = Unbundle(w225) -> (w224:dbl[], w223:dbl[])
        n85 = Array Size(array=w224) -> (size(s)=w228:i32)
        n86 = Decrement(x=w228) -> (x-1=w231:i32)
        n87 = Multiply(x=w231, y="Interpolation factor (n)") -> (x*y=w229:i32)
        n88 = Add(x=w228, y=w229) -> (x+y=w227:i32)
        n89 = Increment(x="Interpolation factor (n)") -> (x+1=w230:i32)
        n90 = for {
          N: w227 -> [_]
          tunnel: w223 -> [w245]
          tunnel: w224 -> [w239]
          tunnel: [w244] -> w226
          tunnel: "Type of Interpolation" -> [w240]
          tunnel: w230 -> [w242]
          tunnel: [w241] -> w221 mode=indexing
          tunnel: [w238] -> w222 mode=indexing
          i -> [w243]
          n91 = Divide(x=w243, y=w242) -> (x/y=w237:dbl)
          n92 = Interpolate 1D Array(1:w237, 2:w239) -> (0:w238:dbl)
          n93 = case shown="\"Spline\"" w240 {
            tunnel: w238 -> [_ w253 w256 w260]
            tunnel: [w247 w252 w254 w262] -> w241
            tunnel: [_ w251 w255 w261] -> w244
            tunnel: w239 -> [_ w250 w257 w263]
            tunnel: w245 -> [w248 w249 w259 w264]
            tunnel: w237 -> [w246 _ _ _]
            frame .."Linear" {
              n94 = Interpolate 1D Array(1:w246, 2:w248) -> (0:w247:dbl)
            }
            frame "Polynomial" {
              n95 = call <vilib>:"Polynomial Interpolation.vi"("x value"=w253, "X"=w250, "Y"=w249) -> ("error"=w251:i32, "interpolation value"=w252:dbl)  [unwired: 1 out]
            }
            frame "Spline" {
              n96 = call <vilib>:"Spline Interpolant.vi"("X"=w257, "Y"=w259) -> ("Interpolant"=w258:dbl[])  [unwired: 2 in, 1 out]
              n97 = call <vilib>:"Spline Interpolation.vi"("x value"=w256, "Interpolant"=w258, "X"=w257, "Y"=w259) -> ("error"=w255:i32, "interpolation value"=w254:dbl)
            }
            frame "Rational".. {
              n98 = call <vilib>:"Rational Interpolation.vi"("x value"=w260, "X"=w263, "Y"=w264) -> ("error"=w261:i32, "interpolation value"=w262:dbl)  [unwired: 1 out]
            }
          }
        }
        n99 = Bundle(w224, w223) -> (w220:cluster{dbl[], dbl[]})  [unwired: 1 in]
        n100 = Bundle(w222, w221) -> (w219:cluster{dbl[], dbl[]})  [unwired: 1 in]
        n101 = call <vilib>:"Error Cluster From Error Code.vi"("error code (0)"=w226) -> ()  [unwired: 8 in, 1 out]
        n102 = for {
          tunnel: w222 -> [w236] mode=indexing
          tunnel: w221 -> [w235] mode=indexing
          tunnel: [w234] -> w217 mode=indexing
          n103 = Bundle(w236, "interpolation value"=w235) -> (w234:cluster{dbl, "interpolation value":dbl})  [unwired: 1 in]
        }
        n104 = Build Array(w220, w219) -> (→"Path":cluster{dbl[], dbl[]}[])
        n105 = call "Set Pure Pursuit Path.vi"("Path"=w217) -> ()  [unwired: 10 in, 1 out]
      }
    }
  }
  n106 = while {
    tunnel: w7 -> [w266]
    stop <- FALSE stop-if-true
    n107 = call "Drive Controller Interactive Check.vi"("Interactive Command In"="Interactive Values", "Default Command"=w266, "Buttons"="Buttons") -> ("Interactive Command Out"=w268:T3, "Trace String"=w269:string, "Schedule"=w270:bool)  [unwired: 6 in]
    n108 = case shown="False" w270 {
      tunnel: [w279 w287] -> w271
      tunnel: [w278 w283] -> w272
      tunnel: w269 -> [_ w285]
      tunnel: w268 -> [_ w284]
      frame False {
        n109 = Tick Count (ms)() -> (millisecond timer value=w282:u32)
        n110 = call "Read Drive Operation.vi"() -> ("Command Info"=w276:T22, "SubSystem Data"=w275:T3)  [unwired: 9 in, 1 out]
        n111 = Unbundle(w275) -> ("Operation"=w280:T4, "Left Setpoint"=w277:dbl)  [unwired: 3 out]
        n112 = Unbundle(w276) -> ("Status"=w279:T6)  [unwired: 2 out]
        n113 = Subtract(x=w282, y=w280) -> (x-y=w281:u32)
        n114 = Bundle(w281, "Left Setpoint"=w277) -> (w278:cluster{u32, "Left Setpoint":dbl})  [unwired: 1 in]
      }
      frame True {
        n115 = call "Drive Command Helper.vi"("Description"=w285, "SubSystem Data"=w284) -> ("Command Info Out"=w286:T22, "Command Timing"=w283:cluster{"Start Time (ms)":u32, "Iterations":i32})  [unwired: 7 in, 1 out]
        n116 = Unbundle(w286) -> ("Status"=w287:T6)  [unwired: 2 out]
      }
    }
    "Status" <- w271
    "Command Timing" <- w272
    n117 = Wait (ms)(milliseconds to wait=u32 20) -> ()  [unwired: 1 out]
  }
  n118 = while {
    tunnel: w2 -> [w292]
    tunnel: w1 -> [w289]
    stop <- FALSE stop-if-true
    # "Tunable PIDF!"
    n119 = feedback #1(T7 {"P Gain"=0.0, "I Gain"=0.0, "D Gain"=0.0, "F Gain"=0.0, "I Zone"=0.0, "Min Output"=0.0, "Max Output"=0.0} ("PID Constants")) -> (w298:T7)
    n120 = Not Equal?(x="PID Constants Drivetrain", y=w298) -> (x != y?=w293:T31)
    n121 = Cluster To Array(cluster=w293) -> (array=w294:bool[])
    n122 = Or Array Elements(Boolean array=w294) -> (logical OR=w296:bool)
    n123 = case shown="True" w296 {
      tunnel: w292 -> [_ w302]
      tunnel: "PID Constants Drivetrain" -> [_ w301]
      tunnel: [w299 w301] -> w297
      tunnel: w298 -> [w299 _]
      tunnel: w289 -> [_ w300]
      frame False {
      }
      frame True {
        n124 = call <vilib>:"Spark MAX Set PIDF Constants.vi"("PID Constants"=w301, "MotorControlDeviceRef"=w302) -> ()  [unwired: 8 in, 2 out]
        n125 = call <vilib>:"Spark MAX Set PIDF Constants.vi"("PID Constants"=w301, "MotorControlDeviceRef"=w300) -> ()  [unwired: 8 in, 2 out]
      }
    }
    n126 = feedback-in #1(w297) -> ()
    n127 = Wait (ms)(milliseconds to wait=u32 100) -> ()  [unwired: 1 out]
  }
  n128 = node-c288(w8) -> ()  [unwired: 1 out]
